vi "test_Setup_Testenvironment.vi"(8 "error in":errorcluster, 11 "device selection":enum16{"monochromator", "CCD", "SCD"}(ring)) -> (0 "error out":errorcluster, 2 "device open for communication?":bool, 3 "GenericDevice.lvclass":refnum<class "GenericDevice.lvclass">)   [LabVIEW 2023]
uses:
  Source/Classes/GenericDevice/GenericDevice.lvclass
  Source/Classes/Mono/Monochromator.lvclass
  Source/Libraries/DeviceManager/DeviceManager.lvlib
  C:/Projects/Horiba/horiba-labview-sdk/Source/Classes/GenericDevice/GenericDevice.lvclass
  C:/Projects/Horiba/horiba-labview-sdk/Source/Classes/Mono/Monochromator.lvclass
  Source/Classes/CCD/CCD.lvclass
  C:/Projects/Horiba/horiba-labview-sdk/Source/Classes/CCD/CCD.lvclass
  Source/Classes/SCD/SCD.lvclass
  C:/Projects/Horiba/horiba-labview-sdk/Source/Classes/SCD/SCD.lvclass
panel:
  # "Connector Pane"
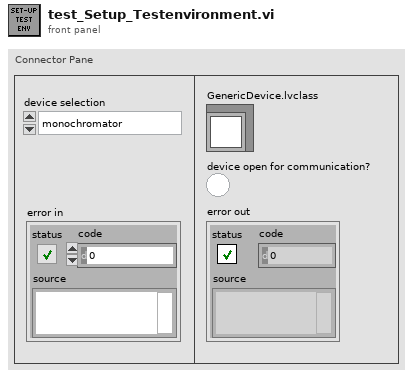
[diagram p1: front panel]
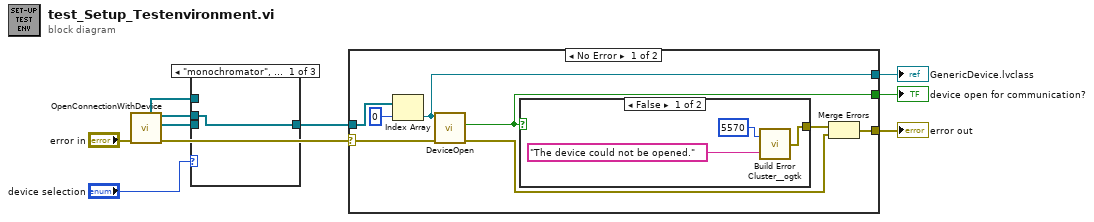
[diagram p0: block diagram]
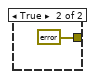
[diagram p4: hidden frame]
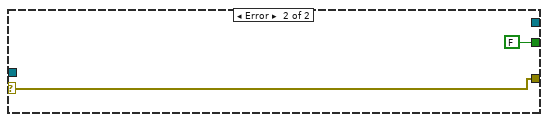
[diagram p5: hidden frame]
diagram:
  n1 = call "OpenConnectionWithDevice.vi"("error in"="error in") -> ("error out"=w10:errorcluster, "CCDs"=w5:refnum<class "CCD.lvclass">[], "Monos"=w6:refnum<class "Monochromator.lvclass">[], "SCDs"=w4:refnum<class "SCD.lvclass">[])  [unwired: 7 in]
  n2 = case shown="\"monochromator\", Default" "device selection" {
    tunnel: w6 -> [w11 _ _]
    tunnel: w5 -> [_ w12 _]
    tunnel: w4 -> [_ _ w13]
    tunnel: [w11 w12 w13] -> w2
    frame "monochromator", Default {
    }
    frame "CCD" {
    }
    frame "SCD" {
    }
  }
  n3 = case shown="No Error" w10 {
    selector: w10 -> [w19 w27]
    tunnel: w2 -> [w21 _]
    tunnel: [w18 w27] -> w8
    tunnel: [w16 FALSE ("CCD open for communication?")] -> w7
    tunnel: [w14 _] -> w1
    frame No Error {
      n4 = Index Array(array=w21, index=0) -> (element=w14:refnum<class "GenericDevice.lvclass">)
      n5 = call-dynamic "DeviceOpen.vi"("error in (no error)"=w19, "GenericDevice in"=w14) -> ("error out"=w15:errorcluster, "device is open?"=w16:bool)  [unwired: 6 in, 2 out]
      n6 = case shown="False" w16 {
        tunnel: [w23 errorcluster {"status"=FALSE, "code"=0, "source"=""} ("error in 2")] -> w17
        frame False {
          n7 = call <userlib>:"Build Error Cluster__ogtk.vi"("String to Prepend to source (\"\")"="The device could not be opened." ("String to Prepend to source (\"\")"), "code"=5570) -> ("error out"=w23:errorcluster)
        }
        frame True {
        }
      }
      n8 = Merge Errors(w17, w15) -> (w18:errorcluster)
    }
    frame Error {
    }
  }
  "error out" <- w8
  "device open for communication?" <- w7
  "GenericDevice.lvclass" <- w1
